vi "ensure_last_waveform_point_0.vi"(11 "Waveform in":waveform(dbl)) -> (3 "Waveform out":waveform(dbl))   [LabVIEW 2019]
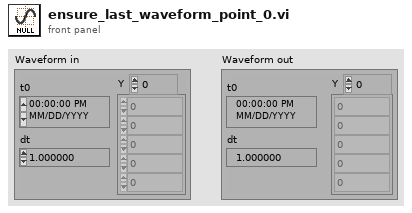
[diagram p1: front panel]
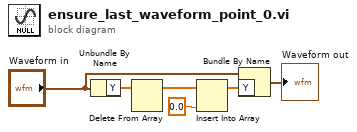
[diagram p0: block diagram]
diagram:
  n1 = Unbundle By Name("Waveform in") -> ("Y"=w6:dbl[])
  n2 = Delete From Array(array=w6) -> (array with subset deleted=w5:dbl[])  [unwired: 2 in, 1 out]
  n3 = Insert Into Array(array=w5, new element=0.0 ("new element/subarray")) -> (w3:dbl[])  [unwired: 1 in]
  n4 = Bundle By Name(cluster="Waveform in", "Y"=w3) -> (→"Waveform out":waveform(dbl))
